vi "Read Data from HW.vi"(11 "Custom Device in":refnum<class "Template.lvclass">) -> (0 "error out":errorcluster, 3 "Custom Device out":refnum<class "Template.lvclass">)   [LabVIEW 2026, in "Template.lvlib" / "Template.lvclass"]
uses:
  Template.lvclass
  Template.lvclass/Template.ctl
  <userlib>/Custom Device Interfaces_v1.lvlibp/CustomDeviceAPI/Custom Device API.lvclass
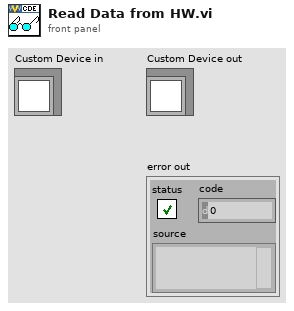
[diagram p1: front panel]
types:
  T1 = cluster{"Data Reference":i32, "Offset":u64, "Length":u64}[]
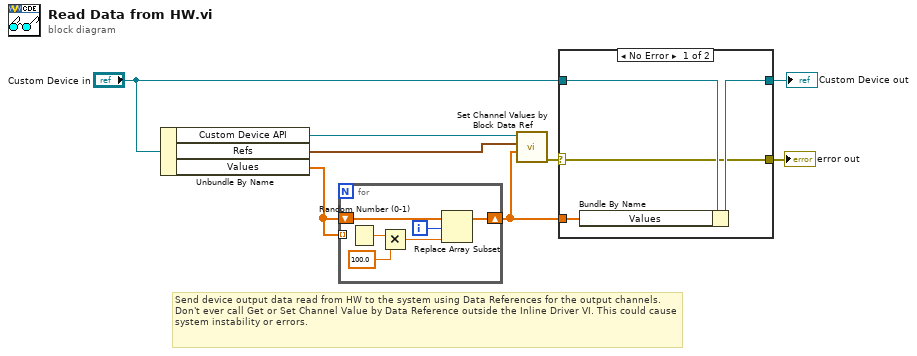
[diagram p0: block diagram]
diagram:
  # "Send device output data read from HW to the system using Data References for the output channels.  Don't ever call Get or Set Channel Value by Data Reference outside the Inline Driver VI. This could cause system instability or errors."
  n1 = Unbundle By Name("Custom Device in") -> ("Custom Device API"=w3:refnum<class "Custom Device API.lvclass">, "Refs"=w2:T1, "Values"=w5:dbl[])
  n2 = for {
    shift-right: [w13] -> w1
    shift-left: w5 -> [w14]
    tunnel: w5 -> [_] mode=indexing
    i -> [w12]
    n3 = Random Number (0-1)() -> (number: 0 to 1=w11:dbl)
    n4 = Multiply(x=w11, y=100.0) -> (x*y=w9:dbl)
    n5 = Replace Array Subset(array=w14, new element=w9, index=w12) -> (w13:dbl[])
  }
  n6 = call-dynamic "Set Channel Values by Block Data Ref.vi"("Values in"=w1, "Block Data Ref in"=w2, "Custom Device API in"=w3) -> ("error out"=w4:errorcluster)  [unwired: 5 in, 3 out]
  n7 = case shown="No Error" w4 {
    selector: w4 -> [w15 w19]
    tunnel: w1 -> [w16 _]
    tunnel: "Custom Device in" -> [w18 w20]
    tunnel: [w17 w20] -> w7
    tunnel: [w15 w19] -> w6
    frame No Error {
      n8 = Bundle By Name(cluster=w18, "Values"=w16) -> (w17:refnum<class "Template.lvclass">)
    }
    frame Error {
    }
  }
  "error out" <- w6
  "Custom Device out" <- w7
